vi "Teleop.vi"(10 "Match Info":T1={"Autonomous Elapsed Seconds"=0.0, "TeleOp Elapsed Seconds"=0.0, "Disabled Elapsed Seconds"=0.0, "Visited Autonomous"=FALSE, "Visited TeleOp"=FALSE, "Visited Disabled"=FALSE, "Autonomous Settings"={"Autonomous Style"=enum."Independent", "VI Refnum"=refnum}}, 11 "Call Context":T2) -> ()   [LabVIEW 2017]
doc: "This VI is called for each TeleOp packet received from the DS where the robot is not disabled. It is often used to read from the joysticks and update I/O or to update setpoints for timed control loops. It should complete and return within 20 milliseconds or it may miss DS packets."
uses:
  <vilib>/Rock Robotics/WPI/DriverStation/WPI_DriverStationDerivedRobotMode.ctl
  <vilib>/Rock Robotics/WPI/DriverStation/WPI_DriverStationMatch Info.ctl
  <vilib>/Rock Robotics/Network Tables/NT Read Boolean.vi
  <vilib>/Rock Robotics/Network Tables/NT Read Number.vi
  <vilib>/Rock Robotics/WPI/Utilities/WPI_GetSetVariantRefNum.vi
  <vilib>/Rock Robotics/Network Tables/NT Write Boolean Array.vi
  <vilib>/Rock Robotics/Network Tables/NT Write Numeric Array.vi
panel:
  out "Lift Bottom":dbl
  out "Lift Top":dbl
  out "Sample Slider 0":dbl(slide) scale=0.0..5.0
  out "Sample Boolean 1":bool
  out "Sample Boolean 0":bool
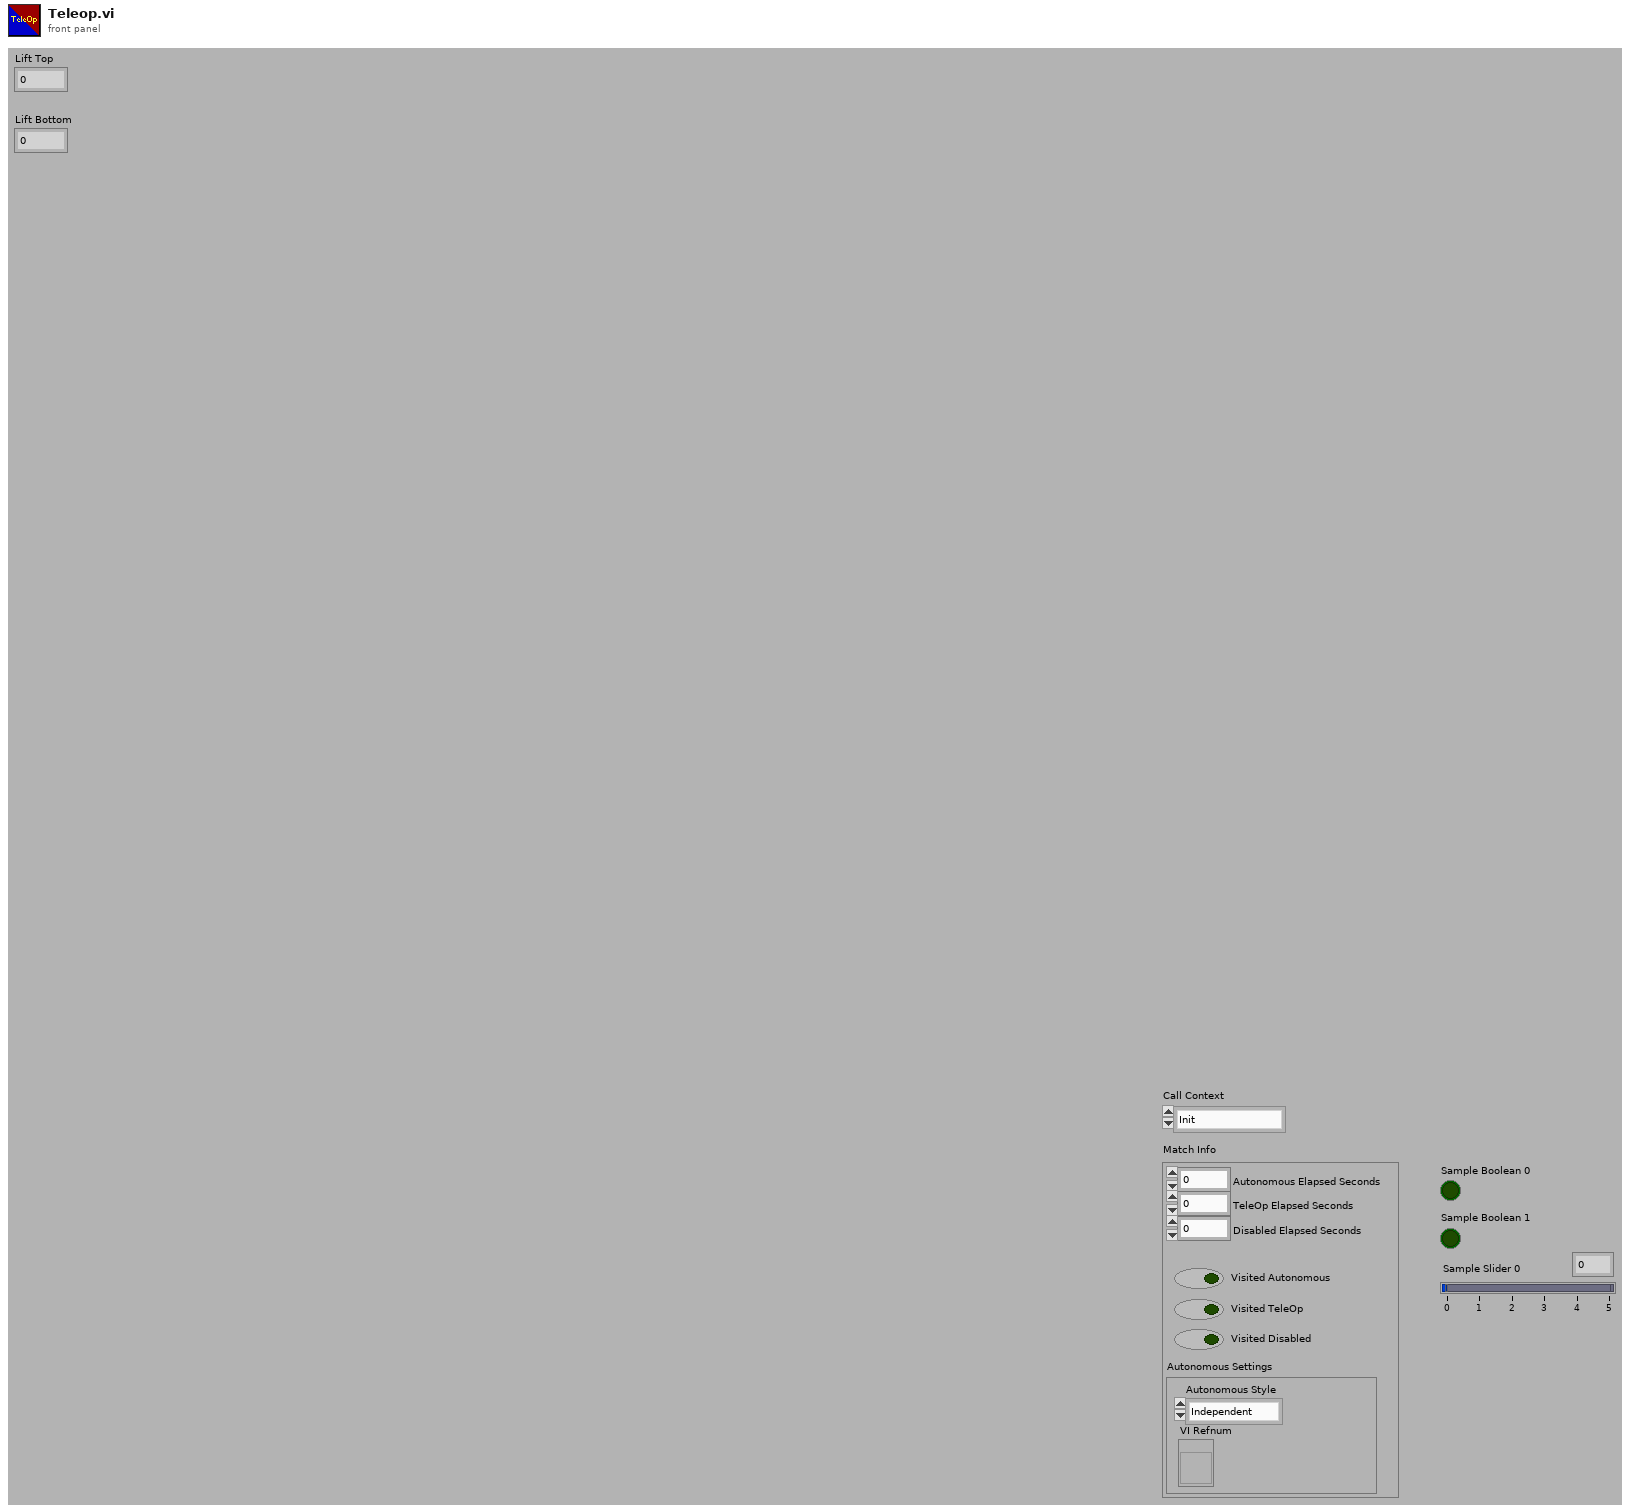
[diagram p1: front panel]
types:
  T1 = typedef "WPI_DriverStationMatch Info.ctl" = cluster{"Autonomous Elapsed Seconds":dbl, "TeleOp Elapsed Seconds":dbl, "Disabled Elapsed Seconds":dbl, "Visited Autonomous":bool, "Visited TeleOp":bool, "Visited Disabled":bool, "Autonomous Settings":cluster{"Autonomous Style":enum16{"Iterative", "Independent"}, "VI Refnum":refnum<vi>}}
  T2 = typedef "WPI_DriverStationDerivedRobotMode.ctl" = enum16{"Init", "Execute", "Stop"}
  T3 = typedef "WPI_JoystickDevRef.ctl" = cluster{"Device":T4}
  T4 = typedef "WPI_JoystickDeviceEnum.ctl" = enum16{"USB 0", "USB 1", "USB 2", "USB 3", "USB 4", "USB 5"}
  T5 = cluster{"Buttons[0]":bool, "Buttons[1]":bool, "Buttons[2]":bool, "Buttons[3]":bool, "Buttons[4]":bool, "Buttons[5]":bool, "Buttons[6]":bool, "Buttons[7]":bool, "Buttons[8]":bool}
  T6 = typedef "WPI_DigitalInputDevRef.ctl" = cluster{"DevStatus":errorcluster, "DIO Channel":T7}
  T7 = typedef "FPGA_DIOChannel.ctl" = enum8{"DIO 0", "DIO 1", "DIO 2", "DIO 3", "DIO 4", "DIO 5", "DIO 6", "DIO 7", "DIO 8", "DIO 9", "DIO MXP 0", "DIO MXP 1", "DIO MXP 2", "DIO MXP 3", "DIO MXP 4", "DIO MXP 5", "DIO MXP 6", "DIO MXP 7", "DIO MXP 8", "DIO MXP 9", "DIO MXP 10", "DIO MXP 11", "DIO MXP 12", "DIO MXP 13", "DIO MXP 14", "DIO MXP 15", "SPI Port CS1", "SPI Port CS2", "SPI Port CS3", "SPI Port MISO", "SPI Port MOSI", "Invalid"}
  T8 = typedef "WPI_RobotDriveDevRef.ctl" = cluster{"DevStatus":errorcluster, "Motors[]":T9[], "Square Inputs":bool, "Max Output":dbl}
  T9 = typedef "WPI_MotorControlDeviceRef.ctl" = cluster{"DeviceStatus":errorcluster, "Type":T10, "PWM":cluster{"PWM Channel":T11, "DeadBand":T12}, "CAN":cluster{"Device Number":u8, "SetOutput VI Ref":variant, "GetOutput VI Ref":variant, "Enable VI Ref":variant, "Disable VI Ref":variant, "Data":variant}, "Invert":bool, "DIO PWM":cluster{"PWM \"Enable\" Channel":T11, "DIOChannel":T7, "PWM Rate":dbl}}
  T10 = typedef "WPI_MotorControlType.ctl" = enum16{"PWM", "CAN", "DIO PWM"}
  T11 = typedef "FPGA_DIOPWMChannel.ctl" = enum8{"PWM 0", "PWM 1", "PWM 2", "PWM 3", "PWM 4", "PWM 5", "PWM 6", "PWM 7", "PWM 8", "PWM 9", "PWM MXP 0", "PWM MXP 1", "PWM MXP 2", "PWM MXP 3", "PWM MXP 4", "PWM MXP 5", "PWM MXP 6", "PWM MXP 7", "PWM MXP 8", "PWM MXP 9", "Invalid"}
  T12 = typedef "WPI_PWMDeadband.ctl" = cluster{"Name":string, "maxPositivePwm":i32, "minPositivePwm":i32, "centerPwm":i32, "maxNegativePwm":i32, "minNegativePwm":i32, "angularRange":u16}
  T13 = cluster{"Axes[0]":dbl, "Axes[1]":dbl, "Axes[2]":dbl, "Axes[3]":dbl, "Axes[4]":dbl, "Axes[5]":dbl, "Axes[6]":dbl, "Axes[7]":dbl, "Axes[8]":dbl}
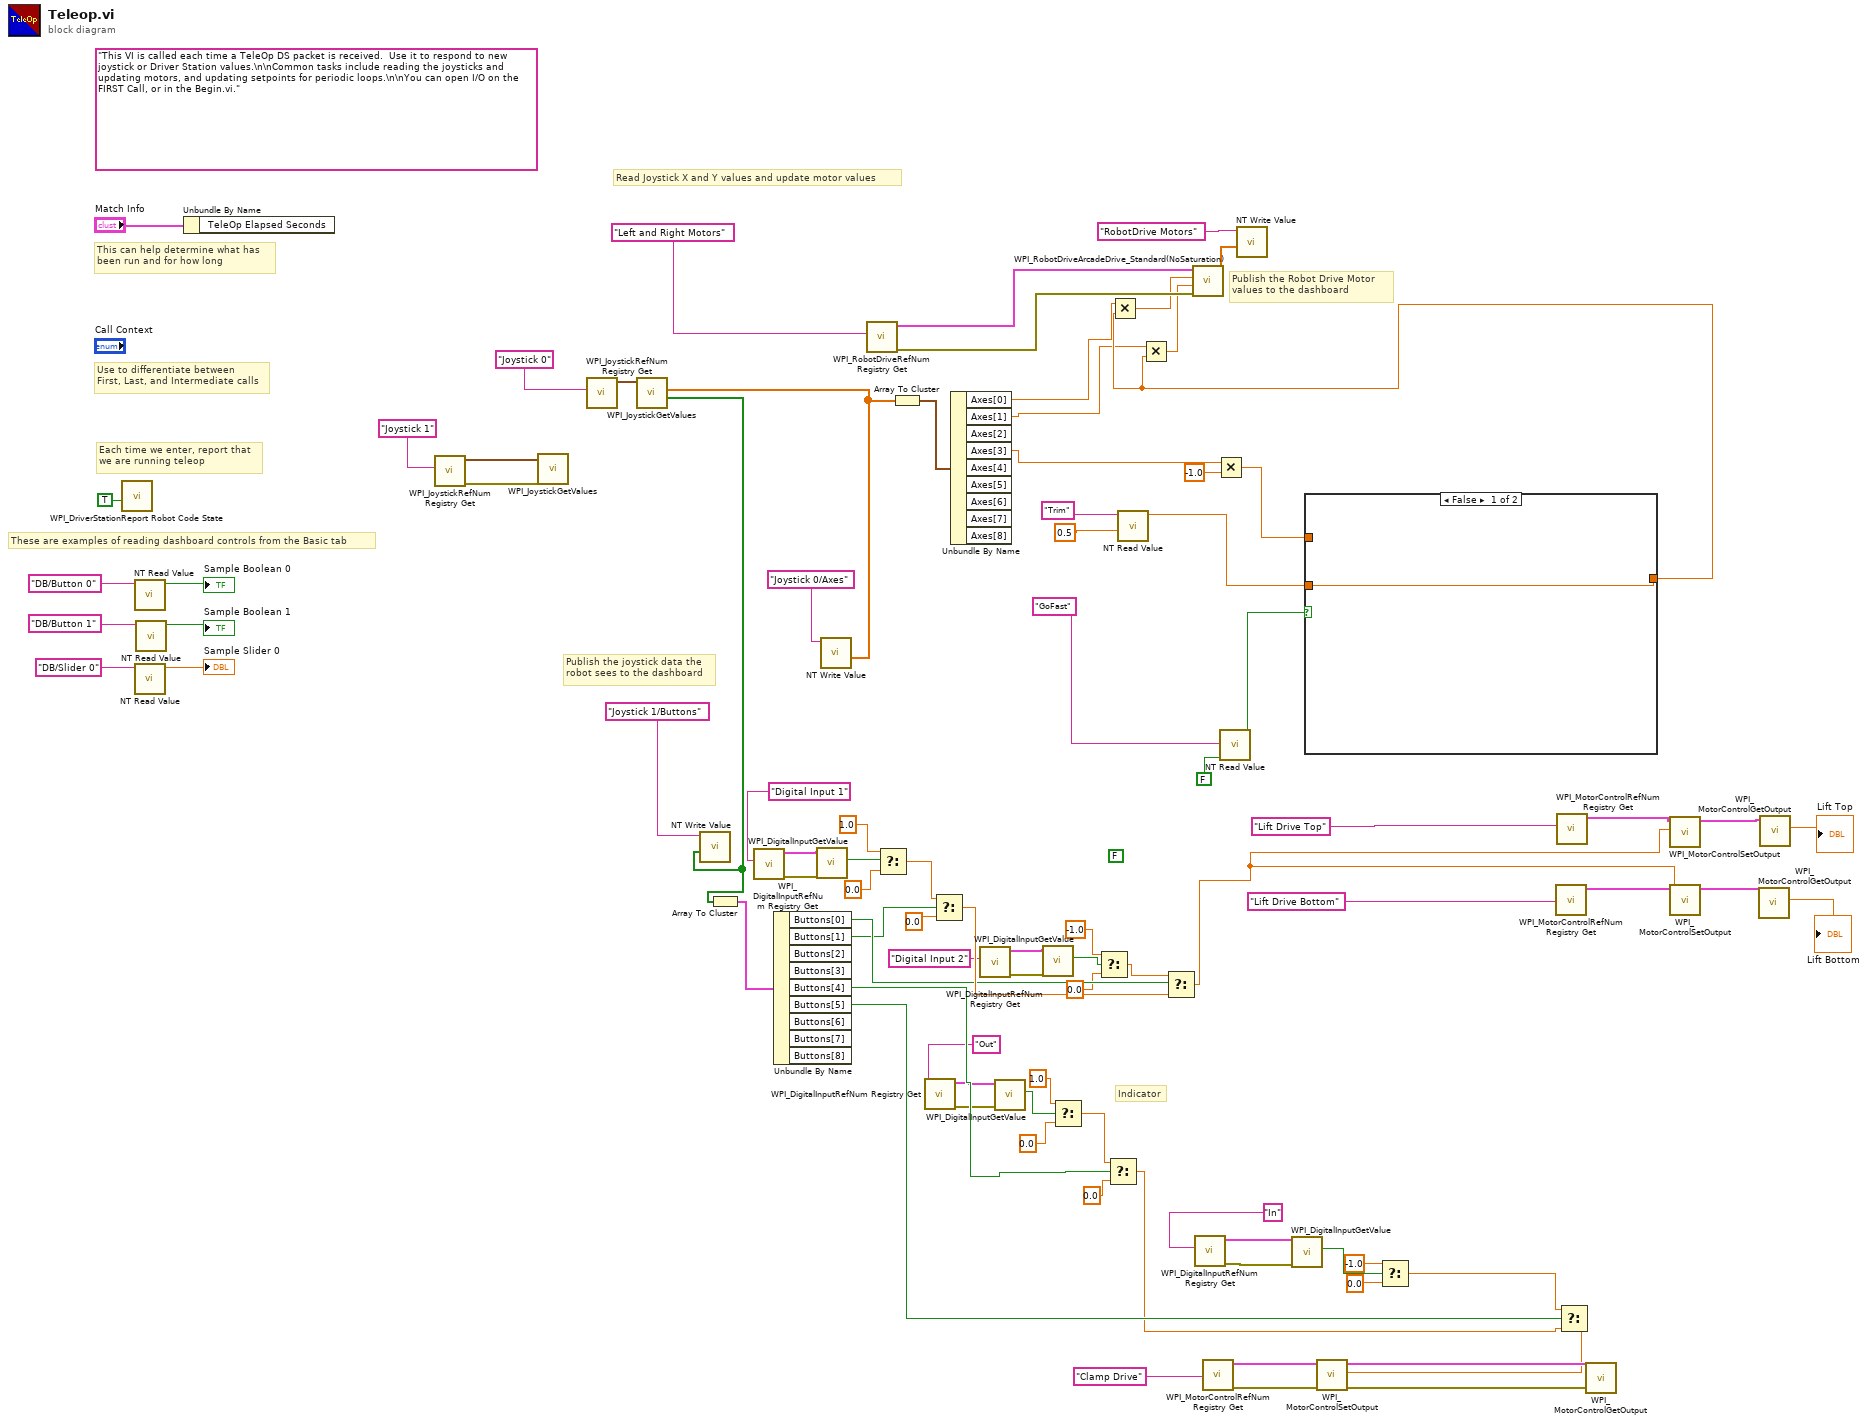
[diagram p0: block diagram]
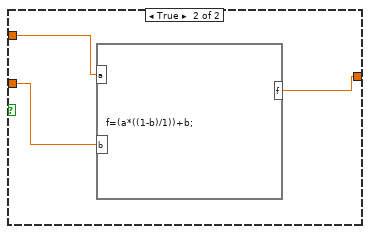
[diagram p2: hidden frame]
diagram:
  (unwired) FALSE ("Default Value")
  (unwired) "This VI is called each time a TeleOp DS packet is received.  Use it to respond to new joystick or Driver Station values.\n\nCommon tasks include reading the joysticks and updating motors, and updating setpoints for periodic loops.\n\nYou can open I/O on the FIRST Call, or in the Begin.vi."
  # "Indicator"
  # "Publish the Robot Drive Motor\nvalues to the dashboard"
  # "Publish the joystick data the\nrobot sees to the dashboard"
  # "Read Joystick X and Y values and update motor values"
  # "These are examples of reading dashboard controls from the Basic tab"
  # "Each time we enter, report that\nwe are running teleop"
  # "Use to differentiate between\nFirst, Last, and Intermediate calls"
  # "This can help determine what has\nbeen run and for how long"
  n1 = call <vilib>:"WPI_DriverStationReport Robot Code State.vi"("TeleOp"=TRUE ("Autonomous")) -> ()  [unwired: 10 in, 1 out]
  n2 = call-poly <vilib>:"NT Read Value.vi"("Name"="DB/Button 0" ("refnum name")) -> ("Boolean"=→"Sample Boolean 0":bool)  [unwired: 9 in, 1 out]
  n3 = call-poly <vilib>:"NT Read Value.vi"("Name"="DB/Slider 0" ("refnum name")) -> ("Numeric"=→"Sample Slider 0":dbl)  [unwired: 9 in, 1 out]
  n4 = call-poly <vilib>:"NT Read Value.vi"("Name"="DB/Button 1" ("refnum name")) -> ("Boolean"=→"Sample Boolean 1":bool)  [unwired: 9 in, 1 out]
  n5 = Unbundle By Name("Match Info") -> ()  [unwired: 1 out]
  n6 = call <vilib>:"WPI_JoystickRefNum Registry Get.vi"("refnum name"="Joystick 1") -> ("error out"=w16:errorcluster, "JoystickDevRef"=w52:T3)  [unwired: 9 in]
  n7 = call <vilib>:"WPI_JoystickGetValues.vi"("error in (no error)"=w16, "JoystickDevRef"=w52) -> ()  [unwired: 5 in, 5 out]
  n8 = call <vilib>:"WPI_JoystickRefNum Registry Get.vi"("refnum name"="Joystick 0") -> ("JoystickDevRef"=w79:T3)  [unwired: 1 in, 9 out]
  n9 = call <vilib>:"WPI_JoystickGetValues.vi"("JoystickDevRef"=w79) -> ("Buttons"=w6:bool[], "Axes"=w57:dbl[])  [unwired: 6 in, 3 out]
  n10 = call-poly <vilib>:"NT Write Value.vi"("Boolean Array"=w6, "Name"="Joystick 1/Buttons") -> ()  [unwired: 9 in, 1 out]
  n11 = Array To Cluster(array=w6) -> (cluster=w58:T5)
  n12 = call <vilib>:"WPI_DigitalInputRefNum Registry Get.vi"("refnum name"="Digital Input 1") -> ("error out"=w34:errorcluster, "DigitalInputDevRef"=w35:T6)  [unwired: 9 in]
  n13 = Unbundle By Name(w58) -> ("Buttons[0]"=w53:bool, "Buttons[1]"=w31:bool, "Buttons[4]"=w28:bool, "Buttons[5]"=w30:bool)  [unwired: 5 out]
  n14 = call <vilib>:"WPI_DigitalInputGetValue.vi"("error in (no error)"=w34, "DigitalInputDevRef"=w35) -> ("Value"=w33:bool)  [unwired: 7 in, 2 out]
  n15 = call-poly <vilib>:"NT Write Value.vi"("Numeric Array"=w57, "Name"="Joystick 0/Axes") -> ()  [unwired: 9 in, 1 out]
  n16 = call <vilib>:"WPI_RobotDriveRefNum Registry Get.vi"("refnum name"="Left and Right Motors") -> ("error out"=w55:errorcluster, "RobotDriveDevRef"=w80:T8)  [unwired: 1 in, 8 out]
  n17 = Select(t=1.0, s=w33, f=0.0) -> (s? t:f=w44:dbl)
  n18 = Array To Cluster(array=w57) -> (cluster=w56:T13)
  n19 = call <vilib>:"WPI_DigitalInputRefNum Registry Get.vi"("refnum name"="Out") -> ("error out"=w18:errorcluster, "DigitalInputDevRef"=w27:T6)  [unwired: 9 in]
  n20 = Select(t=w44, s=w31, f=0.0) -> (s? t:f=w64:dbl)
  n21 = Unbundle By Name(w56) -> ("Axes[0]"=w5:dbl, "Axes[1]"=w4:dbl, "Axes[3]"=w2:dbl)  [unwired: 6 out]
  n22 = call <vilib>:"WPI_DigitalInputRefNum Registry Get.vi"("refnum name"="Digital Input 2") -> ("error out"=w38:errorcluster, "DigitalInputDevRef"=w39:T6)  [unwired: 9 in]
  n23 = call <vilib>:"WPI_DigitalInputGetValue.vi"("error in (no error)"=w18, "DigitalInputDevRef"=w27) -> ("Value"=w25:bool)  [unwired: 7 in, 2 out]
  n24 = call <vilib>:"WPI_DigitalInputGetValue.vi"("error in (no error)"=w38, "DigitalInputDevRef"=w39) -> ("Value"=w37:bool)  [unwired: 7 in, 2 out]
  n25 = Select(t=1.0, s=w25, f=0.0) -> (s? t:f=w22:dbl)
  n26 = Select(t=-1.0, s=w37, f=0.0) -> (s? t:f=w45:dbl)
  n27 = Select(t=w22, s=w28, f=0.0) -> (s? t:f=w19:dbl)
  n28 = call-poly <vilib>:"NT Read Value.vi"("Default Value"=0.5, "Name"="Trim" ("refnum name")) -> ("Numeric"=w10:dbl)  [unwired: 8 in, 1 out]
  n29 = Select(t=w45, s=w53, f=w64) -> (s? t:f=w65:dbl)
  n30 = call <vilib>:"WPI_DigitalInputRefNum Registry Get.vi"("refnum name"="In") -> ("error out"=w49:errorcluster, "DigitalInputDevRef"=w51:T6)  [unwired: 9 in]
  n31 = call <vilib>:"WPI_MotorControlRefNum Registry Get.vi"("refnum name"="Clamp Drive") -> ("error out"=w63:errorcluster, "MotorControlDevRef"=w61:T9)  [unwired: 9 in]
  n32 = Multiply(x=w2, y=-1.0) -> (x*y=w3:dbl)
  n33 = call-poly <vilib>:"NT Read Value.vi"("Default Value"=FALSE, "Name"="GoFast" ("refnum name")) -> ("Boolean"=w11:bool)  [unwired: 8 in, 1 out]
  n34 = call <vilib>:"WPI_DigitalInputGetValue.vi"("error in (no error)"=w49, "DigitalInputDevRef"=w51) -> ("Value"=w47:bool)  [unwired: 7 in, 2 out]
  n35 = case shown="False" w11 {
    tunnel: [w90 w93] -> w8
    tunnel: w10 -> [w90 w92]
    tunnel: w3 -> [_ w91]
    frame False {
    }
    frame True {
      n36 = formula code="f=(a*((1-b)/1))+b;"("a"=w91, "b"=w92) -> ("f"=w93:dbl)
    }
  }
  n37 = Multiply(x=w5, y=w8) -> (x*y=w7:dbl)
  n38 = Multiply(x=w4, y=w8) -> (x*y=w9:dbl)
  n39 = call <vilib>:"WPI_RobotDriveArcadeDrive_Standard(NoSaturation).vi"("error in (no error)"=w55, "Y axis value"=w9, "X axis value"=w7, "RobotDriveDevRef"=w80) -> ("Motor Values"=w76:dbl[])  [unwired: 7 out]
  n40 = call-poly <vilib>:"NT Write Value.vi"("Numeric Array"=w76, "Name"="RobotDrive Motors") -> ()  [unwired: 9 in, 1 out]
  n41 = Select(t=-1.0, s=w47, f=0.0) -> (s? t:f=w20:dbl)
  n42 = call <vilib>:"WPI_MotorControlRefNum Registry Get.vi"("refnum name"="Lift Drive Bottom") -> ("MotorControlDevRef"=w70:T9)  [unwired: 9 in, 1 out]
  n43 = call <vilib>:"WPI_MotorControlRefNum Registry Get.vi"("refnum name"="Lift Drive Top") -> ("MotorControlDevRef"=w71:T9)  [unwired: 9 in, 1 out]
  n44 = Select(t=w20, s=w30, f=w19) -> (s? t:f=w46:dbl)
  n45 = call <vilib>:"WPI_MotorControlSetOutput.vi"("error in (no error)"=w63, "Output"=w46, "MotorControlDevRef"=w61) -> ("error out"=w60:errorcluster, "MotorControlDevRef"=w62:T9)  [unwired: 6 in, 1 out]
  n46 = call <vilib>:"WPI_MotorControlGetOutput.vi"("error in"=w60, "MotorControlDevRef"=w62) -> ()  [unwired: 7 in, 3 out]
  n47 = call <vilib>:"WPI_MotorControlSetOutput.vi"("Output"=w65, "MotorControlDevRef"=w71) -> ("MotorControlDevRef"=w72:T9)  [unwired: 7 in, 2 out]
  n48 = call <vilib>:"WPI_MotorControlSetOutput.vi"("Output"=w65, "MotorControlDevRef"=w70) -> ("MotorControlDevRef"=w73:T9)  [unwired: 7 in, 2 out]
  n49 = call <vilib>:"WPI_MotorControlGetOutput.vi"("MotorControlDevRef"=w73) -> ("Output"=→"Lift Bottom":dbl)  [unwired: 8 in, 2 out]
  n50 = call <vilib>:"WPI_MotorControlGetOutput.vi"("MotorControlDevRef"=w72) -> ("Output"=→"Lift Top":dbl)  [unwired: 8 in, 2 out]
